vi "Camera Loop.vi"() -> ()   [LabVIEW 2012]
uses:
  <vilib>/Platform/TimedLoop/XDataNode/timing_clust.ctl
  <vilib>/Platform/TimedLoop/XDataNode/nitl_modes.ctl
  <vilib>/Platform/TimedLoop/XDataNode/wakeup.ctl
  <vilib>/platform/TimedLoop/XDataNode/XDataNode.xnode
  <vilib>/Platform/TimedLoop/XDataNode/XDNodeRunTimeDep.lvlib
panel:
  out "Image Type":T1 items=["Grayscale (U8)", "Grayscale (I16)", "Grayscale (SGL)", "Complex (CSG)", "RGB (U32)", "HSL (U32)", "RGB (U64)", "Grayscale (U16)"]
  out "Y Resolution":i32
  out "X Resolution":i32
  out "RGB":u32[][](graph)
  out "HSV":u32[][](graph)
  out "Image Index":dbl
  out "Time Stamp":timestamp
  in  "Record Button":bool
  in  "Save File Path":path
  out "Gauge":cluster{dbl, dbl}(knob) scale=0.0..50.0
  out "Error Out":errorcluster
  in  "Error In":errorcluster
  in  "Stop (F)":bool
  out "Right Image":T2(plugin-control)
  out "Left Image":T2(plugin-control)
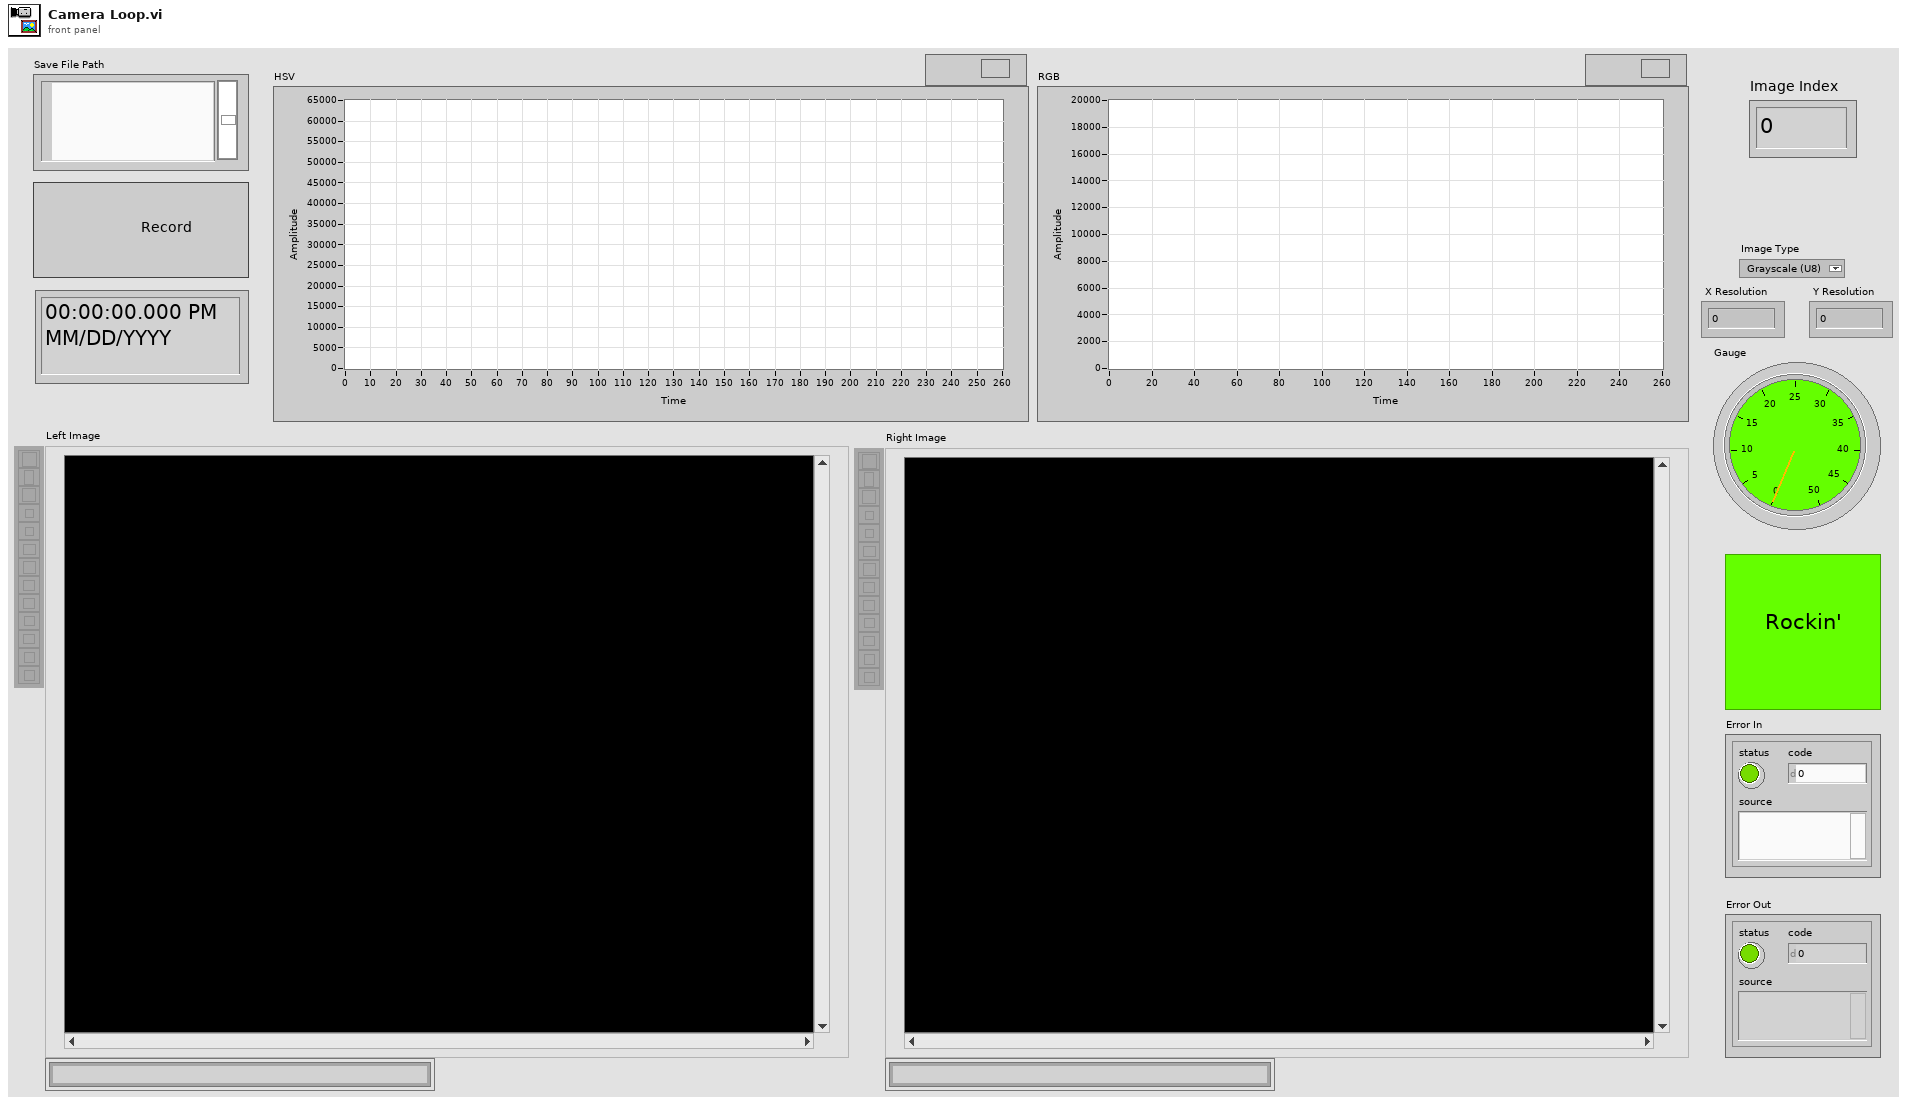
[diagram p1: front panel]
types:
  T1 = typedef "Image Type" = u32
  T2 = typedef "IMAQ Image.ctl" = refnum<image>
  T3 = typedef "XDNodeRunTimeDep.lvlib/timing_clust.ctl" = cluster{"Expected End [f-1]":u64, "Actual End [f-1]":u64, "Finished Late? [f-1]":bool, "Expected End [i-1]":u64, "Actual End [i-1]":u64, "Finished Late? [i-1]":bool, "Expected Start [i]":u64, "Actual Start [i]":u64, "Expected Start [f]":u64, "Actual Start [f]":u64, "Source Name":string, "Structure Name":string, "Period":i64, "Deadline":i64, "Offset":i64, "Start":i64, "Priority":i32, "Timeout":i32, "Mode":T4, "Wakeup Reason":T5, "Error":errorcluster, "Source Type":string, "Secondary Source Type":string, "Global End Time":u64, "Global Start Time":u64, "Frame Duration":u64, "Iteration Duration":u64, "Assigned CPU":i32, "I/O Scan Engine Mode":u32}
  T4 = typedef "XDNodeRunTimeDep.lvlib/nitl_modes.ctl" = enum32{"No Change", "Process missed periods, maintain original phase", "Discard missed periods, maintain original phase", "Process missed periods, ignore original phase", "Discard missed periods, ignore original phase"}
  T5 = typedef "XDNodeRunTimeDep.lvlib/wakeup.ctl" = enum32{"Normal", "Aborted", "Asynchronous wakeup", "Timing source error", "Timed loop error", "Timeout"}
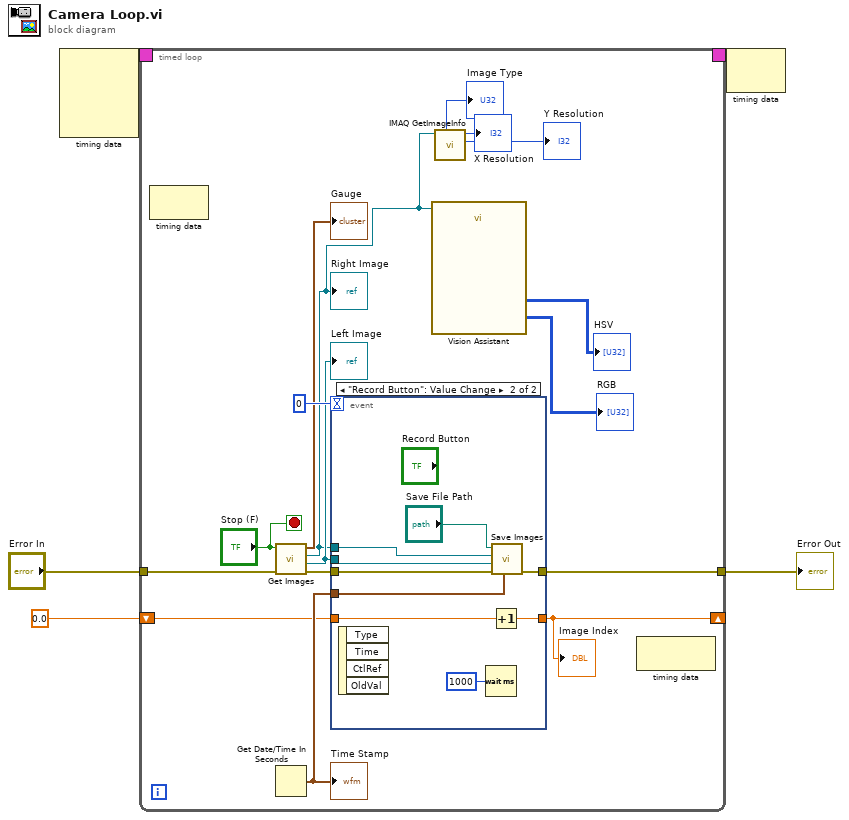
[diagram p0: block diagram]
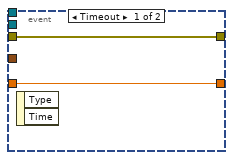
[diagram p2: hidden frame]
diagram:
  n1 = node-c288() -> (w5:T3)  [unwired: 4 in]
  n2 = timed-loop {
    timing: w5 -> [_]
    timing-out: [_] -> w4
    tunnel: "Error In" -> [w16]
    tunnel: [w20] -> w2
    shift-right: [w18] -> _
    shift-left: 0.0 ("Image Index") -> [w17]
    stop <- "Stop (F)" stop-if-true
    n3 = node-c288() -> ()  [unwired: 1 in, 1 out]
    n4 = call "Get Images.vi"("error in"=w16, "Stop (F)"="Stop (F)") -> ("error out"=w15:errorcluster, "Left Image"=w13:T2, "Right Image"=w9:T2, "Gauge"=→"Gauge":cluster{dbl, dbl})  [unwired: 6 in]
    "Left Image" <- w13
    "Right Image" <- w9
    n5 = Get Date/Time In Seconds() -> (seconds since 1Jan1904=w21:timestamp)
    "Time Stamp" <- w21
    n6 = event shown="[1] \"Record Button\": Value Change" {
      selector: _ -> [_ _]
      dyn-events: _ -> [_ _]
      timeout: 0 -> [_ _]
      tunnel: w21 -> [_ w27]
      tunnel: w15 -> [w23 w31]
      tunnel: [w23 w30] -> w20
      tunnel: [w22 w28] -> w18
      tunnel: w17 -> [w22 w29]
      tunnel: w9 -> [_ w26]
      tunnel: w13 -> [_ w25]
      event Timeout {
        n7 = event-data() -> ()  [unwired: 1 in, 2 out]
      }
      event "Record Button": Value Change {
        n8 = event-data() -> ()  [unwired: 1 in, 4 out]
        n9 = Wait (ms)(milliseconds to wait=u32 1000) -> ()  [unwired: 1 out]
        n10 = Increment(x=w29) -> (x+1=w28:dbl)
        n11 = call "Save Images.vi"("Time Stamp"=w27, "error in (no error)"=w31, "Left Image"=w25, "Right Image"=w26, "Save File Path"="Save File Path") -> ("error out"=w30:errorcluster)  [unwired: 6 in]
      }
    }
    "Image Index" <- w18
    n12 = call "Vision Assistant"("Image In"=w9) -> ("Histogram (Histogram 1)"=→"HSV":u32[][], "Histogram (Histogram 2)"=→"RGB":u32[][])  [unwired: 23 in, 2 out]
    n13 = call "IMAQ GetImageInfo"("Image"=w9) -> ("Y Resolution"=→"Y Resolution":i32, "X Resolution"=→"X Resolution":i32, "Image Type"=→"Image Type":T1)  [unwired: 3 in, 5 out]
    n14 = node-c288() -> ()  [unwired: 1 in, 1 out]
  }
  "Error Out" <- w2
  n15 = node-c288(w4) -> ()  [unwired: 1 out]
